vi "call_fixed_array.vi"(9 "column":u16, 10 "row":u16, 11 "array":u8[](array[numeric])) -> (3 "element":u8)   [LabVIEW 2009]
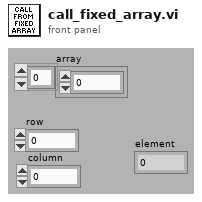
[diagram p1: front panel]
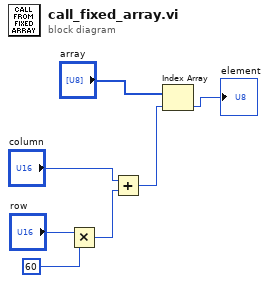
[diagram p0: block diagram]
diagram:
  n1 = Multiply(x="row", y=u16 60 ("row length")) -> (x*y=w5:u16)
  n2 = Add(x="column", y=w5) -> (x+y=w3:u16)
  n3 = Index Array(array="array", index=w3) -> (element=→"element":u8)
